vi "Gestione_Inverter.vi"(6 "Inverter":refnum<vi>, 7 "Stato rpm":refnum<vi>, 8 "Test settings":refnum<vi>, 9 "RS485":refnum<vi>, 10 "Cluster ALARMS":refnum<vi>, 11 "name":string) -> ()   [LabVIEW 2019]
uses:
  Letture inverter.ctl
  Parametri inverter.ctl
  Da TDE TestDrive/Tipi di parametro.ctl
  Set inverter.ctl
  <vilib>/Modbus/subvis/Modbus API/Modbus API.lvclass/Modbus API.ctl
  <vilib>/Modbus/subvis/Transmission Data Unit (ADU)/Transmission Data Unit/Transmission Data Unit.lvclass/Transmission Data Unit.ctl
  <vilib>/Modbus/master/Data Access/Unit ID/Set Unit ID Property.vi
  <vilib>/Modbus/subvis/Transmission Data Unit (ADU)/Transmission Data Unit/Data Access/Unit ID/Write Unit ID.vi
  <vilib>/Modbus/subvis/Modbus API/Read Transmission Data Unit.vi
  <vilib>/Modbus/subvis/Modbus API/Write Transmission Data Unit.vi
  <vilib>/Modbus/master/Modbus Master.lvclass
  C:/Program Files (x86)/National Instruments/LabVIEW 2019/vi.lib/Modbus/subvis/Modbus API/Modbus API.lvclass
  <vilib>/Utility/file.llb/Read From Spreadsheet File (string).vi
  <vilib>/Modbus/master/Create Master Instance (Serial).vi
  <vilib>/Modbus/subvis/Transmission Data Unit (ADU)/Transmission Data Unit/Transmission Data Unit.lvclass
panel:
  in  "SET INVERTER":bool
  in  "Test settings 2":T1 caption="PARAMETRI INVERTER"
  in  "Scelta inverter":T2(radio)=enum."INVERTER 1 \n[7,5kW]"
  out "id":u8
  in  "stop":bool
  out "DRIVE INOM":dbl
  out "Numeric":i32
  out "status":string
  out "output cluster":T3
  out "error out":errorcluster
  # "Caratteristiche motore"
  # "Limiti massimi"
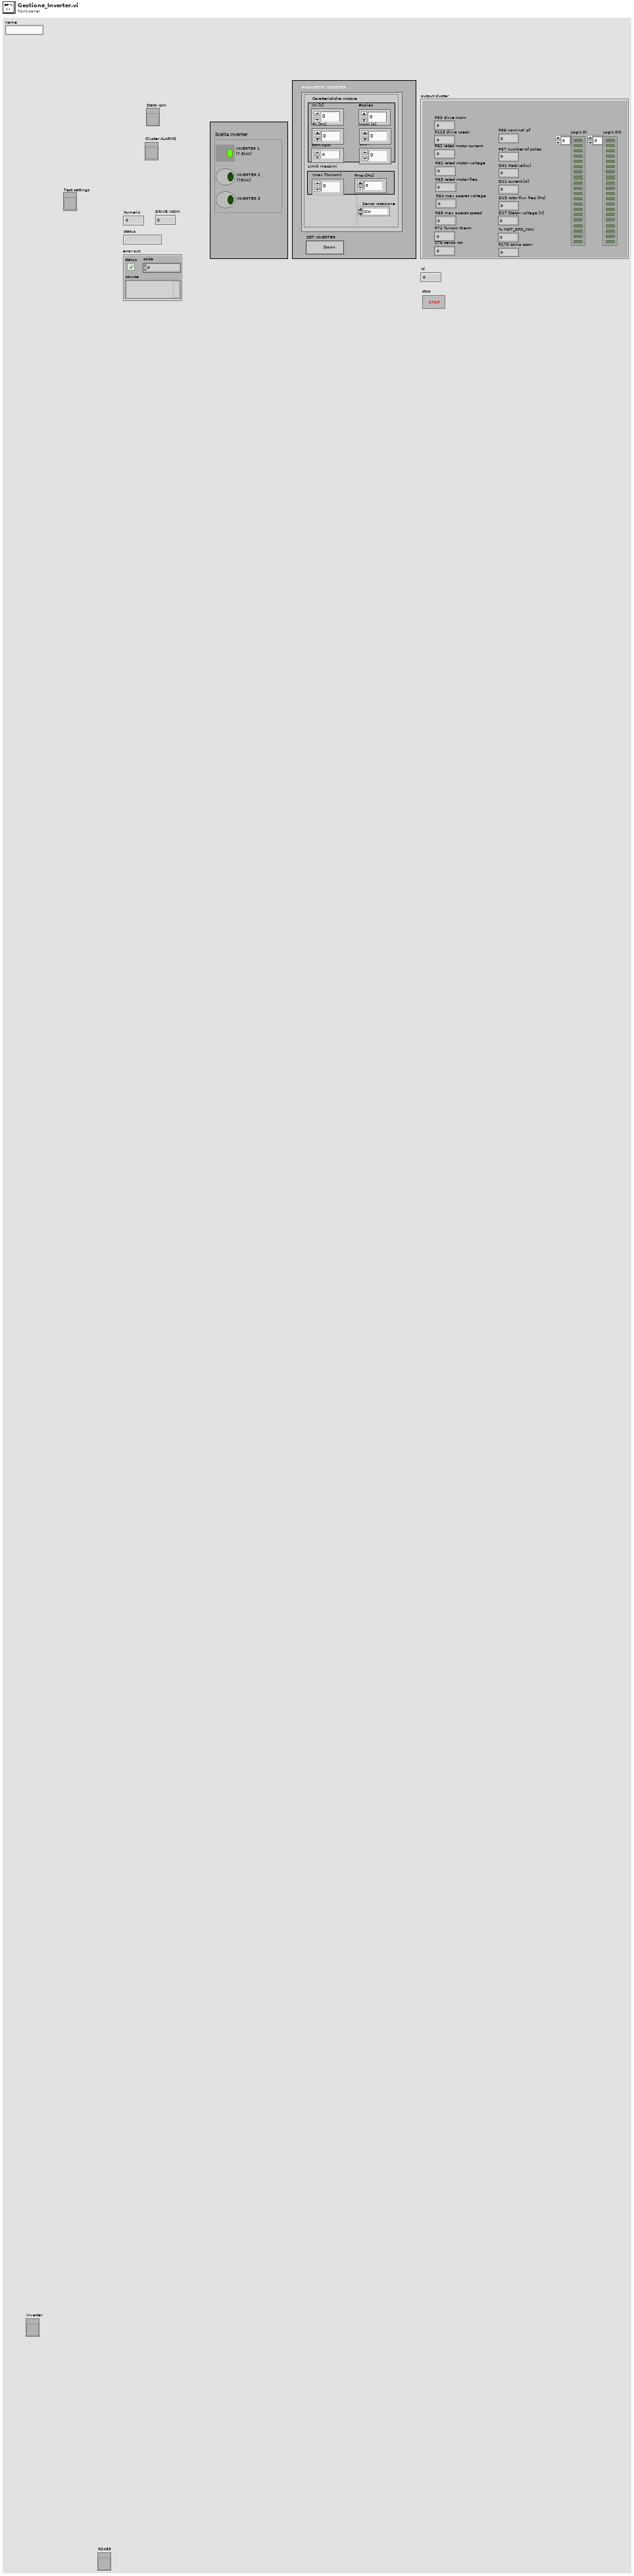
[diagram p1: front panel]
types:
  T1 = typedef "Parametri inverter.ctl" = cluster{"Vn [V]":dbl, "Fn [Hz]":dbl, "CosFi":dbl, "Imax [%Inom]":dbl, "#poles":dbl, "Inom [A]":dbl, "Senso rotazione":enum16{"CW", "CCW"}, "RPM nom":dbl, "Fmax[Hz]":dbl}
  T2 = enum32{"No Selection", "INVERTER 1 \n[7,5kW]", "INVERTER 2 \n[75kW]", "INVERTER 3"}
  T3 = typedef "Letture inverter.ctl" = cluster{"P61 rated motor current":dbl, "P62 rated motor voltage":dbl, "P63 rated motor freq":dbl, "P64 max operat voltage":dbl, "P65 max operat speed":dbl, "P66 nominal pf":dbl, "P67 number of poles":dbl, "D01 Pattiva[kw]":dbl, "D11 current [A]":dbl, "D13 rotor flux freq [Hz]":dbl, "D17 Stator voltage [V]":dbl, "% MOT_SPD_MAX":dbl, "Logic DI":bool[], "Logic DO":bool[], "P71 %inom therm":dbl, "P53 dirve Inom":dbl, "P113 dirve Ipeak":dbl, "C76 senso rot":dbl, "P170 comp scorr":dbl}
  T4 = typedef "Tipi di parametro.ctl" = u16
  T5 = typedef "Set inverter.ctl" = cluster{"F [Hz]":dbl}
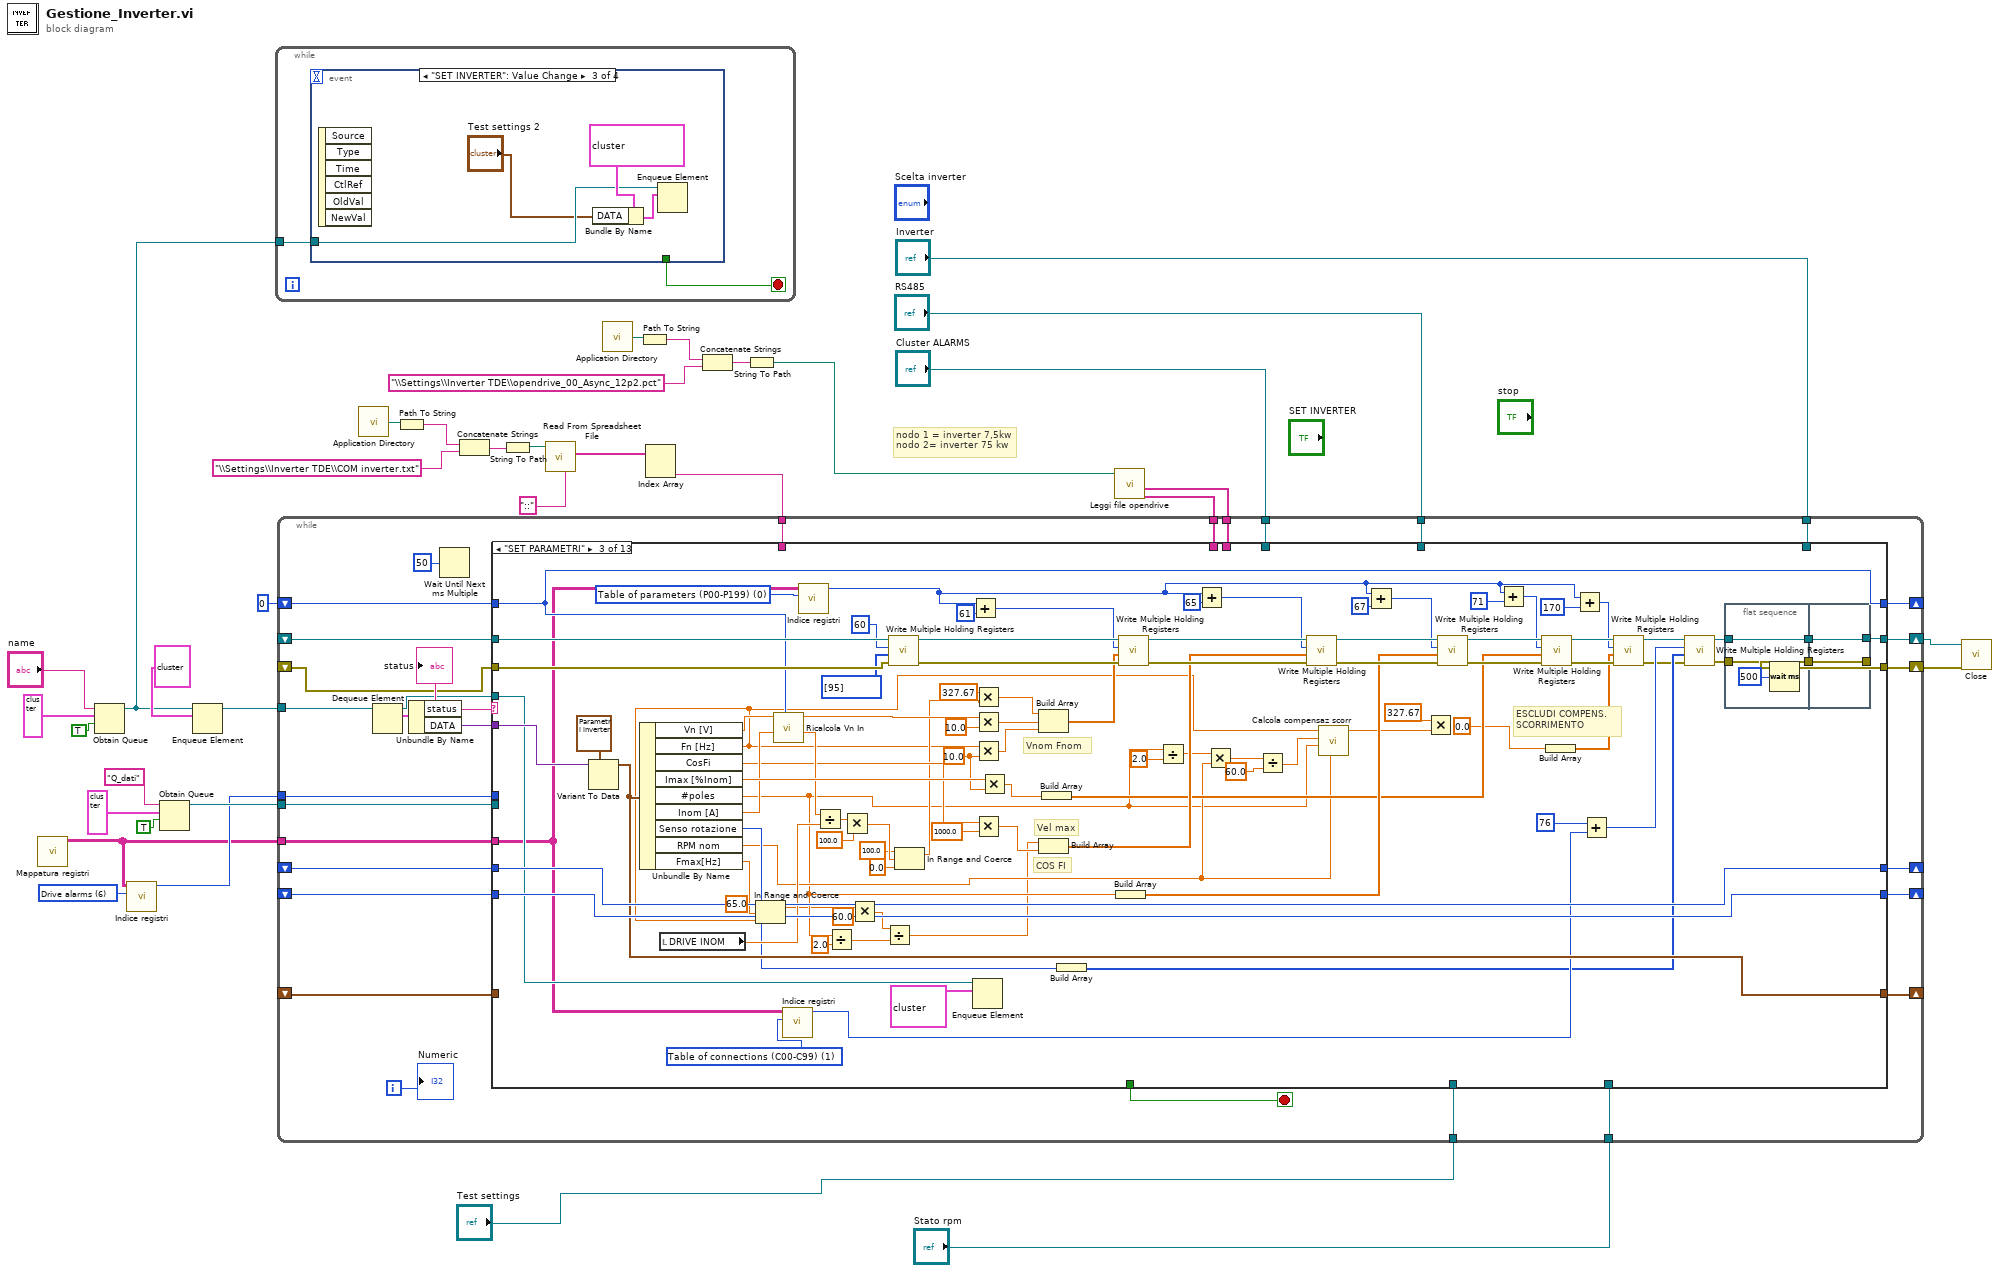
[diagram p0: block diagram]
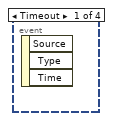
[diagram p2: hidden frame]
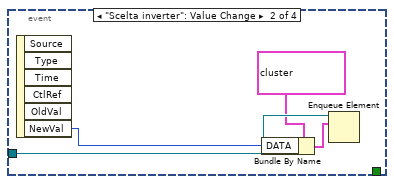
[diagram p3: hidden frame]
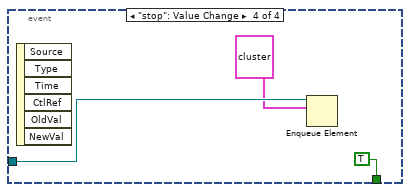
[diagram p4: hidden frame]
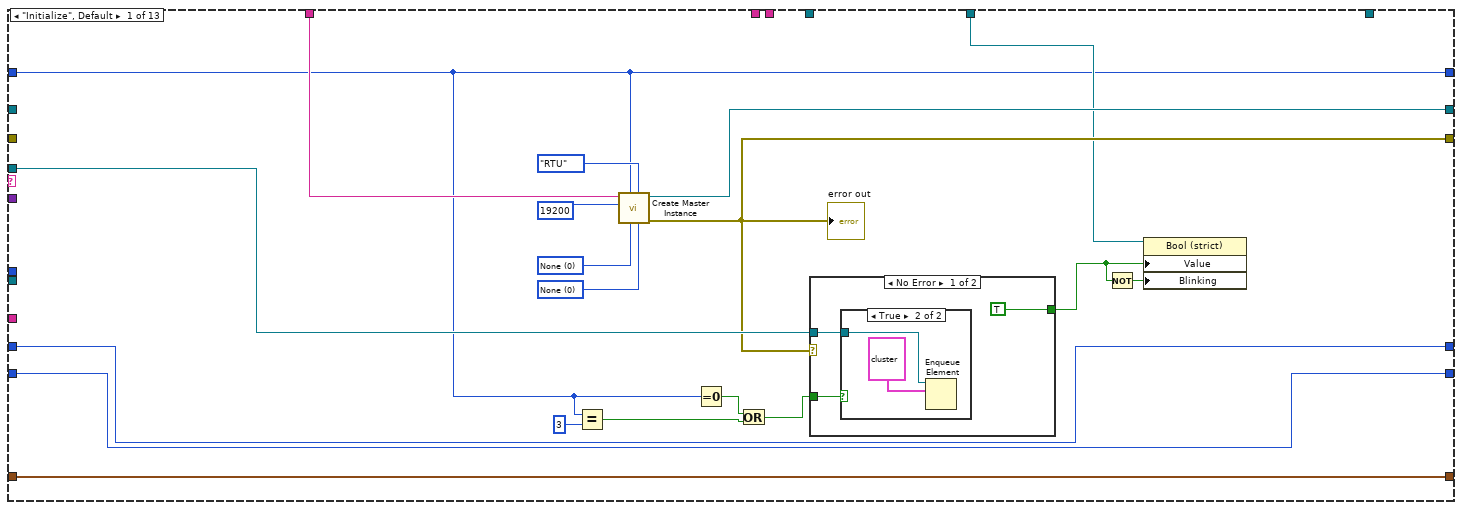
[diagram p5: hidden frame]
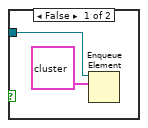
[diagram p6: hidden frame]
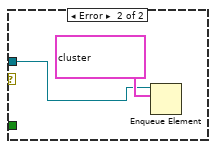
[diagram p7: hidden frame]
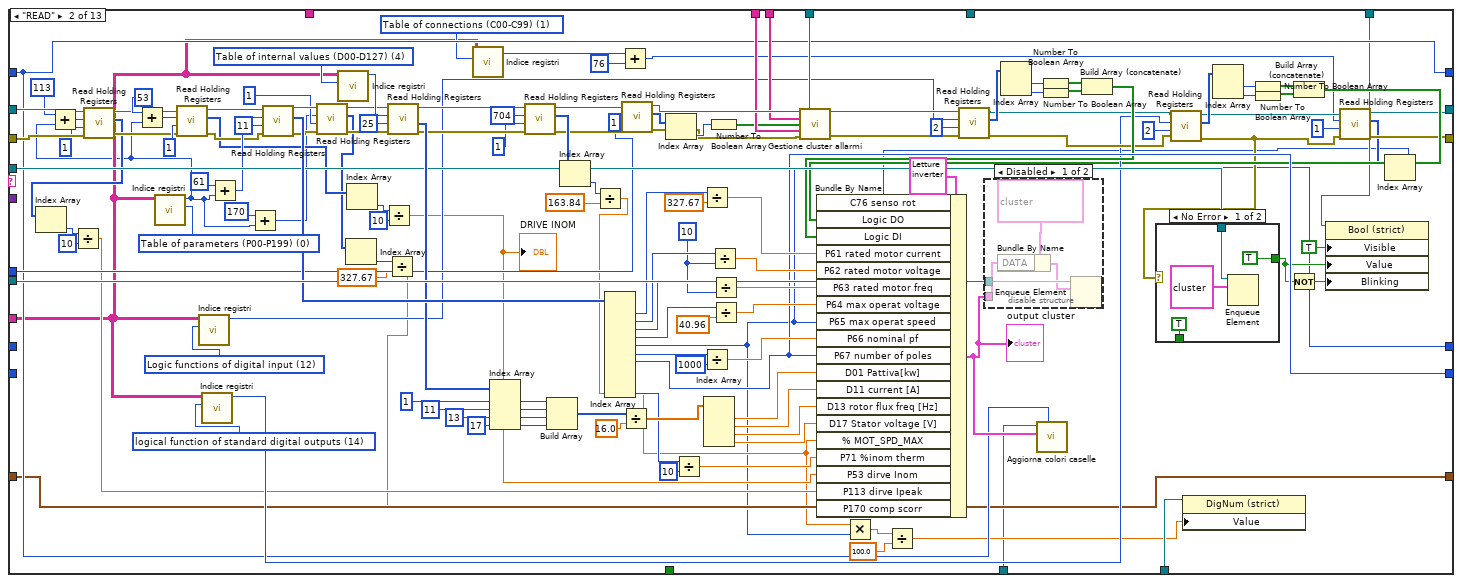
[diagram p8: hidden frame]
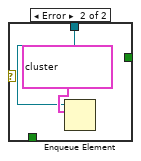
[diagram p10: hidden frame]
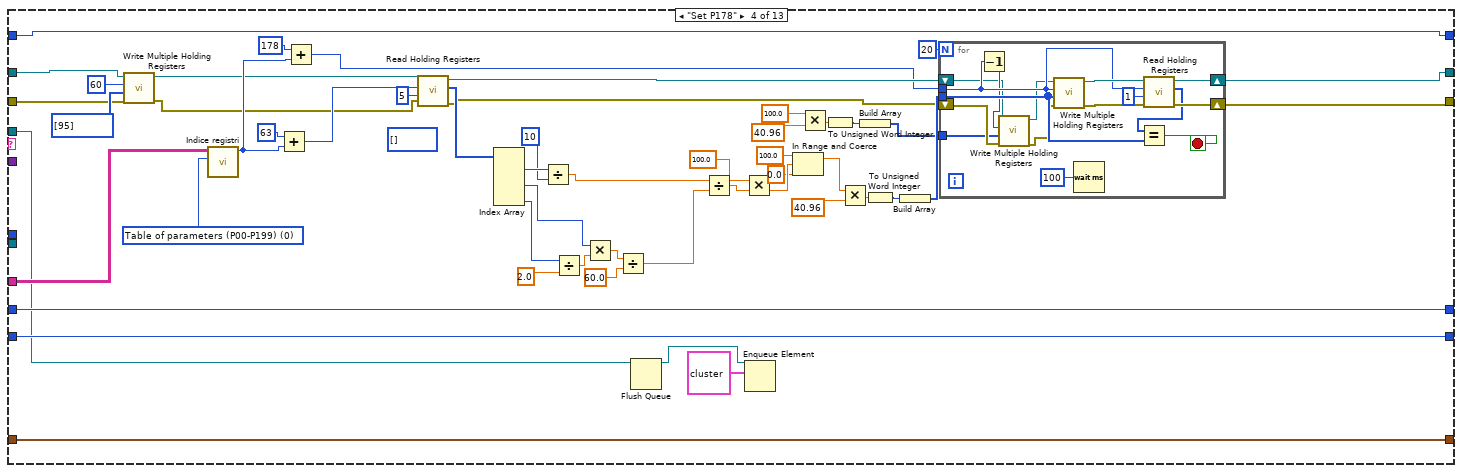
[diagram p11: hidden frame]
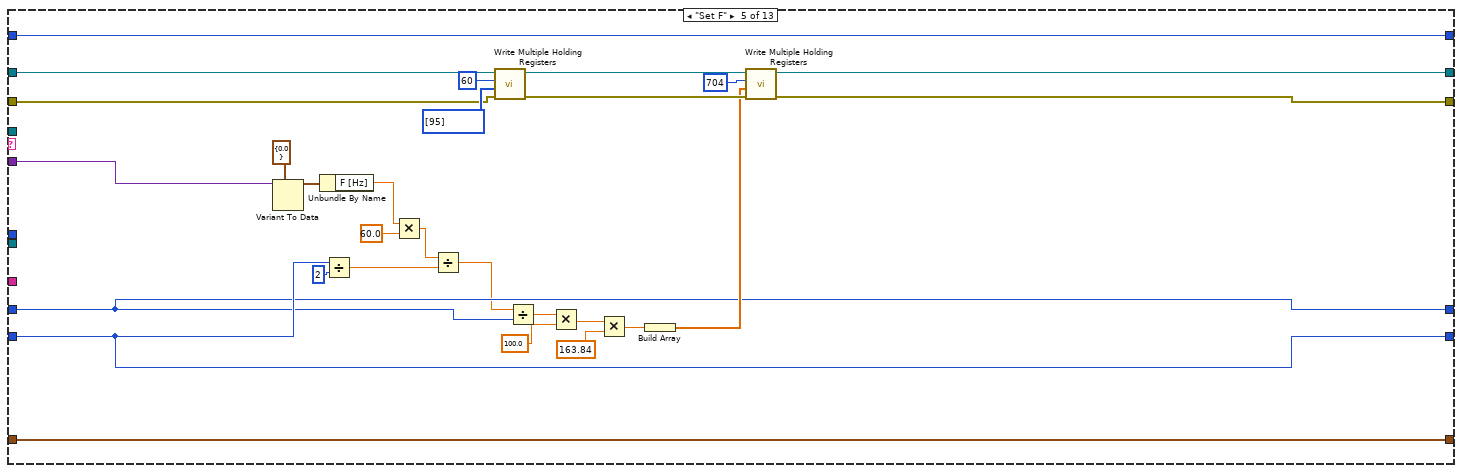
[diagram p12: hidden frame]
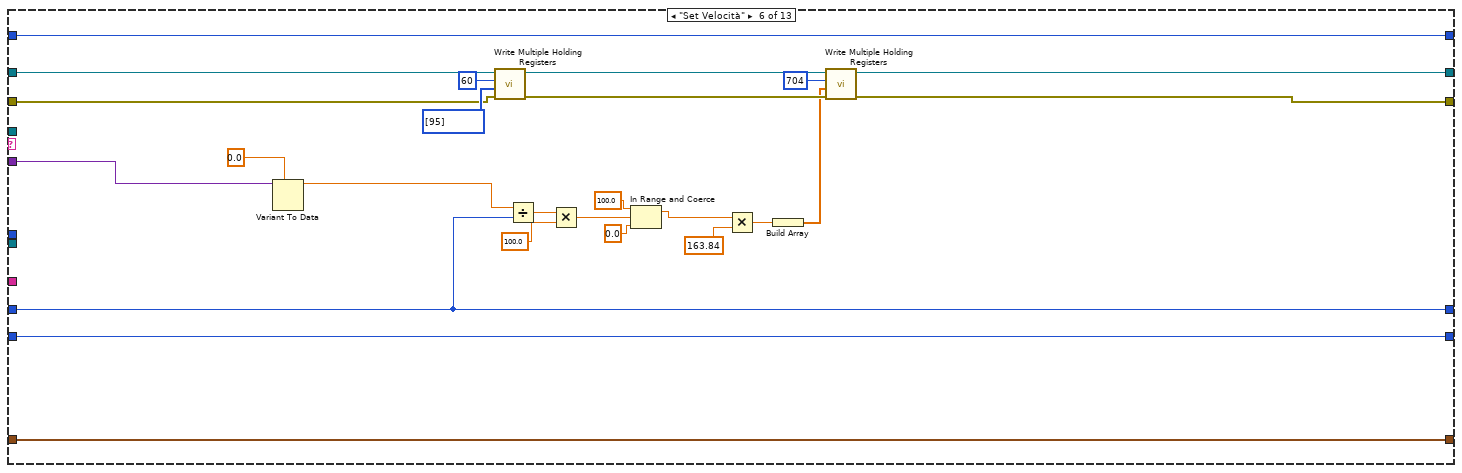
[diagram p13: hidden frame]
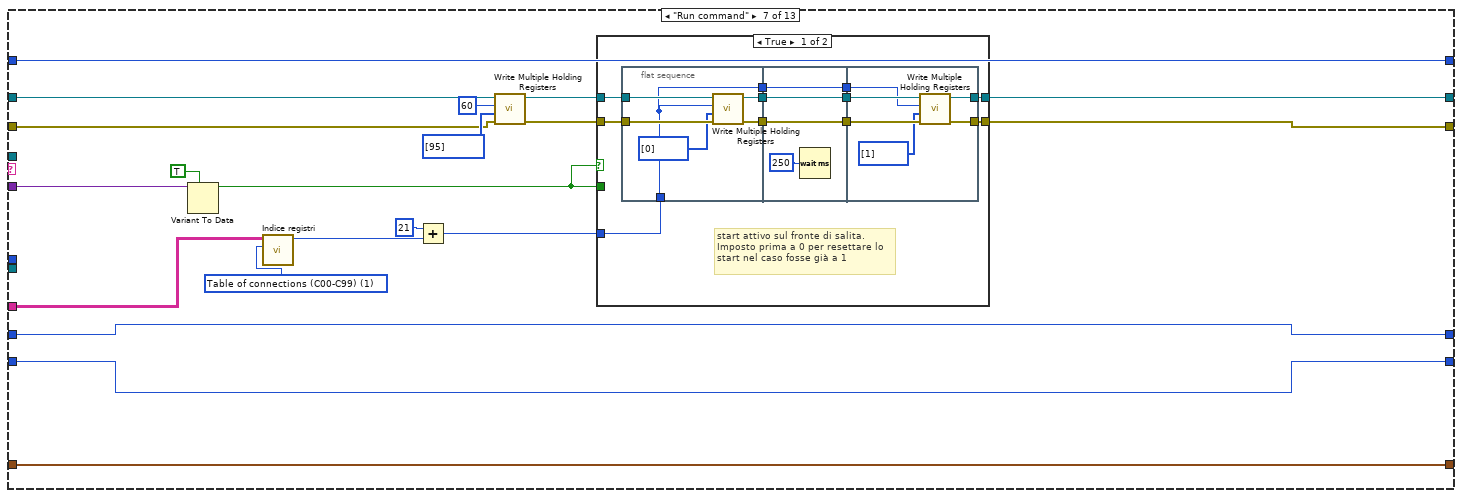
[diagram p14: hidden frame]
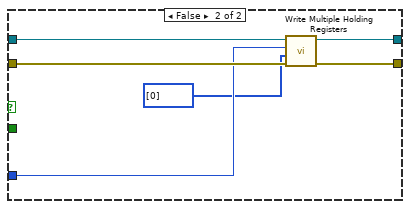
[diagram p15: hidden frame]
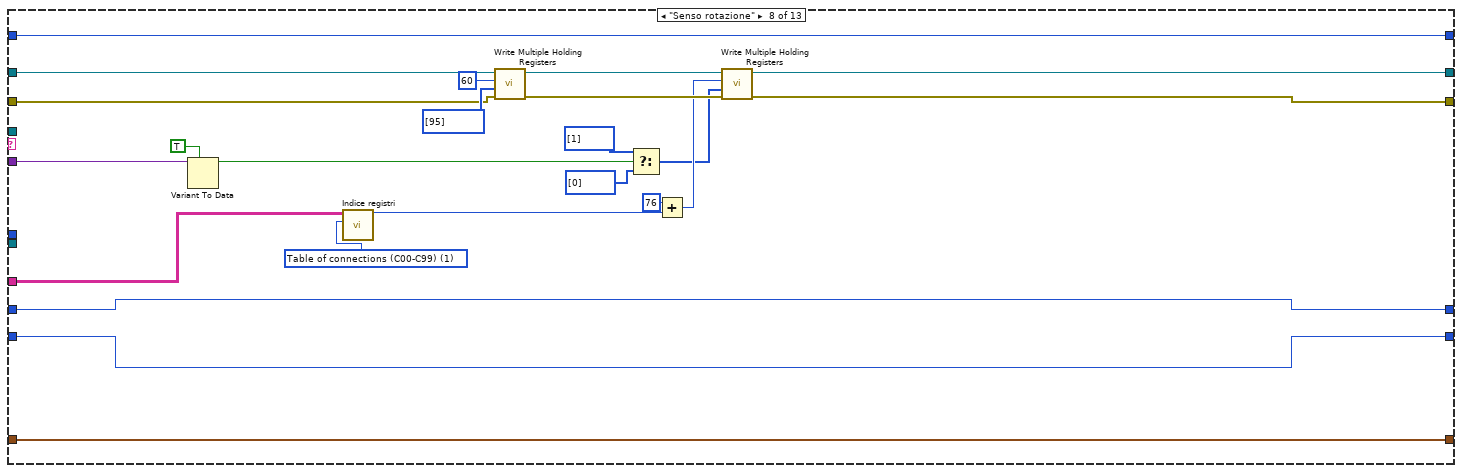
[diagram p16: hidden frame]
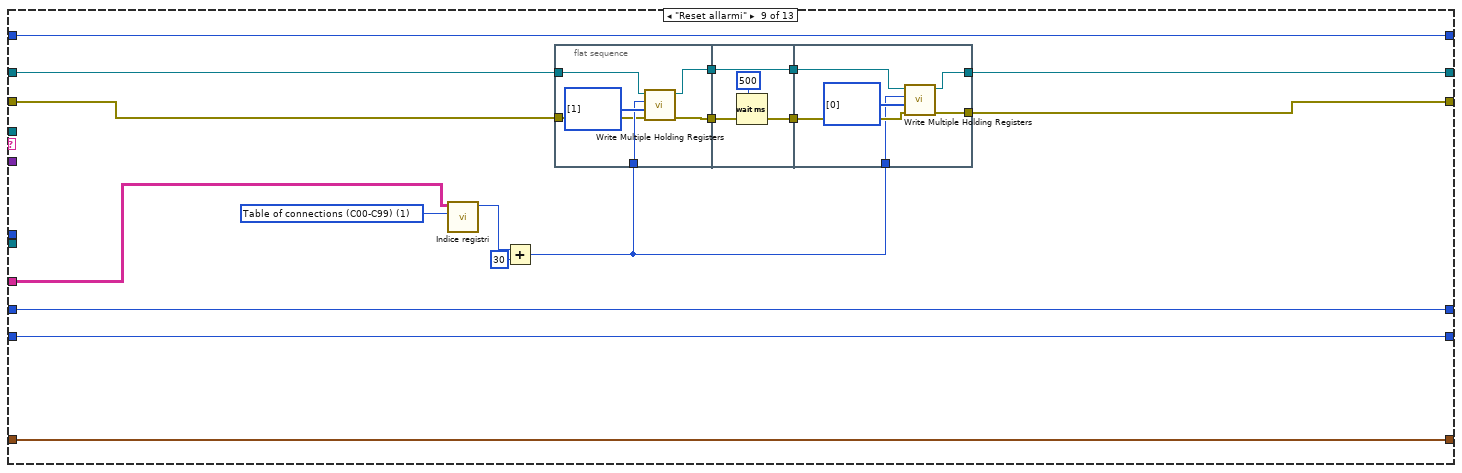
[diagram p17: hidden frame]
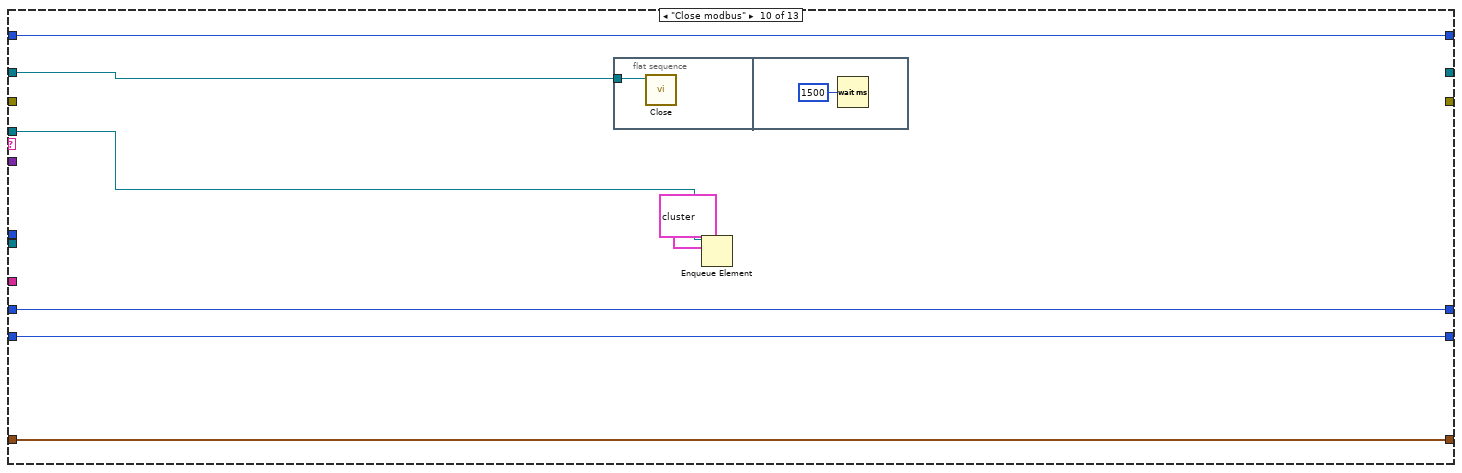
[diagram p18: hidden frame]
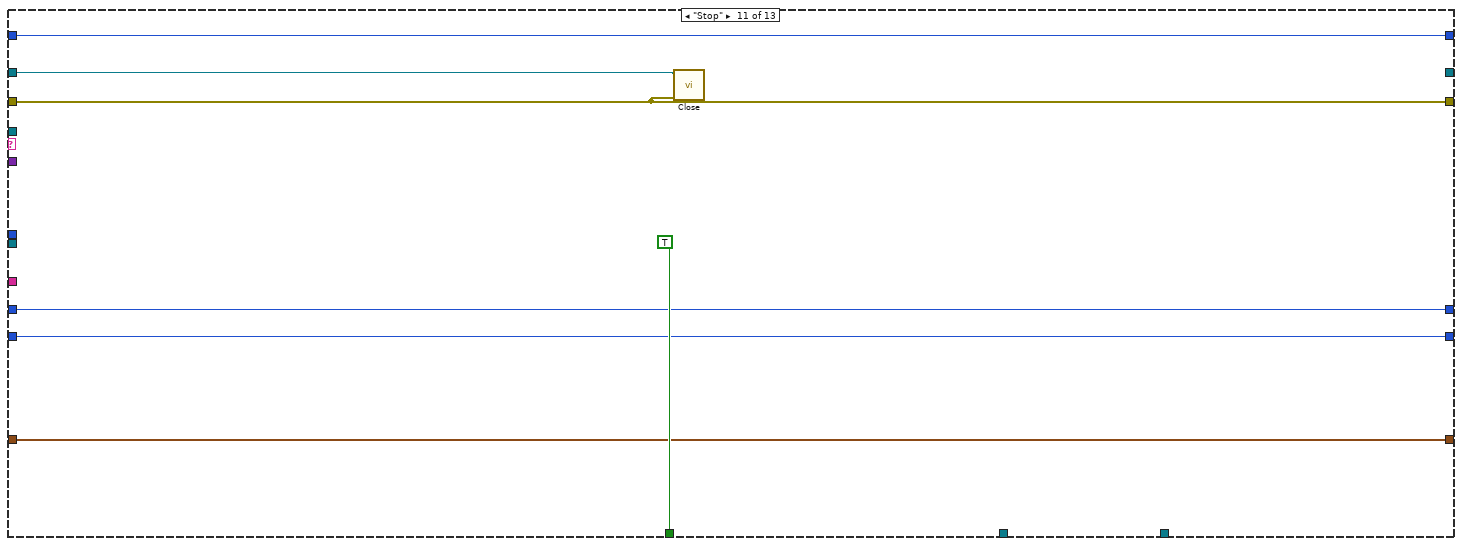
[diagram p19: hidden frame]
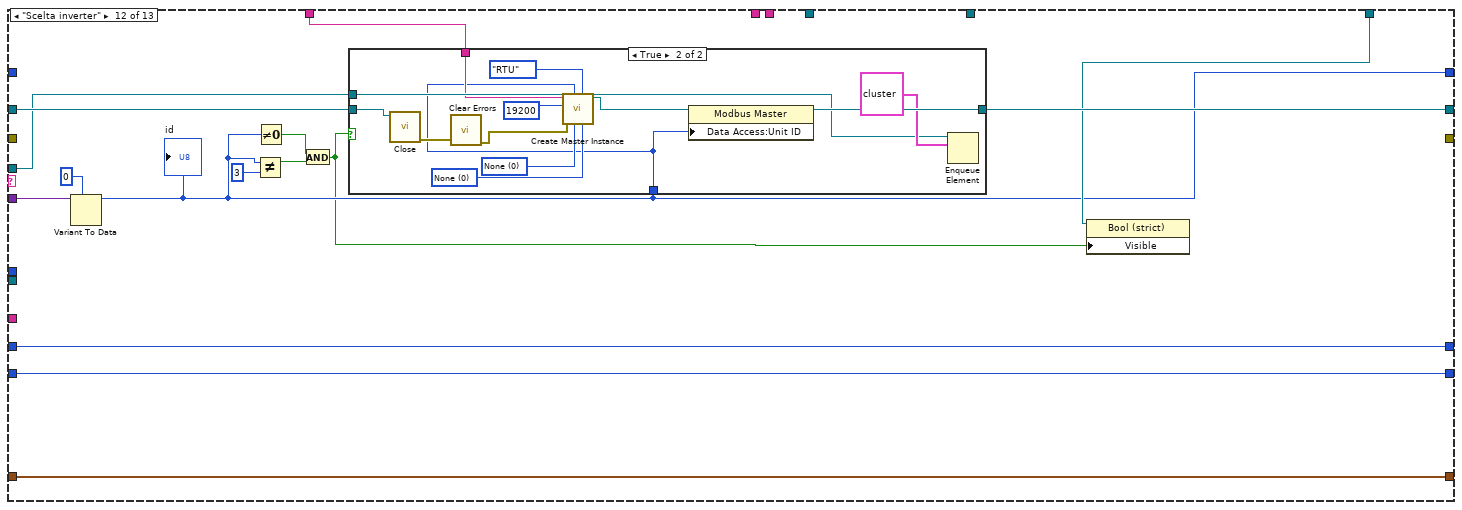
[diagram p20: hidden frame]
diagram:
  w25 = T4 6 items=["Table of parameters (P00-P199)", "Table of connections (C00-C99)", "Table of application parameters (E00-E99)", "Table of expanded application parameters (E100-E600)", "Table of internal values (D00-D127)", "Drive state", "Drive alarms", "Alarm enabling", "Speed reference from fieldbus", "Torque limit from fieldbus", "Torque reference from fieldbus", "Mechanical position read", "Logic functions of digital input", "Logic funtction of digital input from serial c.", "logical function of standard digital outputs", "logic function of application digital output", "Table of parameters formats", "Table of connections formats", "Table of monitor and analog outputs values", "Table of application parameters formats", "Table of internal values formats", "Scorta 1", "Scorta 2", "Scorta 3", "Scorta 4", "Scorta 5", "Scorta 6", "Scorta 7", "Scorta 8", "Scorta 9", "Scorta 10"] ("Lista tipi di parametro")
  # "nodo 1 = inverter 7,5kw\nnodo 2= inverter 75 kw"
  n1 = call "Mappatura registri.vi"() -> ("Mappa registri"=w20:string[][])  [unwired: 11 in]
  n2 = Obtain Queue(name (unnamed)="name", element data type=cluster{"DATA":variant, "status":string} {"DATA"=variant, "status"=""} ("output cluster"), create if not found? (T)=TRUE) -> (queue out=w5:refnum<queue>)  [unwired: 2 in, 2 out]
  n3 = call "Indice registri.vi"("Lista tipi di parametro"=w25, "Mappa registri"=w20) -> ("Registro iniziale"=w24:i32)  [unwired: 7 in, 2 out]
  n4 = Obtain Queue(name (unnamed)="Q_dati", element data type=cluster{"DATA":variant, "status":string} {"DATA"=variant, "status"=""} ("output cluster"), create if not found? (T)=TRUE) -> (queue out=w30:refnum<queue>)  [unwired: 2 in, 2 out]
  n5 = Enqueue Element(queue=w5, element=cluster{"DATA":variant, "status":string} {"DATA"=variant, "status"="IDLE"}) -> (queue out=w28:refnum<queue>)  [unwired: 2 in, 2 out]
  n6 = while {
    tunnel: w5 -> [w38]
    stop <- w37 stop-if-true
    n7 = event shown="[2] \"SET INVERTER\": Value Change" {
      selector: _ -> [_ _ _ _]
      dyn-events: _ -> [_ _ _ _]
      timeout: _ -> [_ _ _ _]
      tunnel: w38 -> [_ w42 w44 w49]
      tunnel: [_ _ _ TRUE] -> w37
      event Timeout {
        n8 = event-data() -> ()  [unwired: 1 in, 3 out]
      }
      event "Scelta inverter": Value Change {
        n9 = event-data() -> ("NewVal"=w39:T2)  [unwired: 1 in, 5 out]
        n10 = Bundle By Name(cluster=cluster{"DATA":variant, "status":string} {"DATA"=variant, "status"="Scelta inverter"} ("element"), "DATA"=w39) -> (w40:cluster{"DATA":variant, "status":string})
        n11 = Enqueue Element(queue=w42, element=w40) -> ()  [unwired: 2 in, 3 out]
      }
      event "SET INVERTER": Value Change {
        n12 = event-data() -> ()  [unwired: 1 in, 6 out]
        n13 = Bundle By Name(cluster=cluster{"DATA":variant, "status":string} {"DATA"=variant, "status"="SET PARAMETRI"} ("element"), "DATA"="Test settings 2") -> (w45:cluster{"DATA":variant, "status":string})
        n14 = Enqueue Element(queue=w44, element=w45) -> ()  [unwired: 2 in, 3 out]
      }
      event "stop": Value Change {
        n15 = event-data() -> ()  [unwired: 1 in, 6 out]
        n16 = Enqueue Element(queue=w49, element=cluster{"DATA":variant, "status":string} {"DATA"=variant, "status"="Stop"}) -> ()  [unwired: 2 in, 3 out]
      }
    }
  }
  n17 = call <vilib>:"Application Directory.vi"() -> ("Application Directory"=w14:path)
  n18 = Path To String(path=w14) -> (string=w15:string)
  n19 = Concatenate Strings(w15, "\\Settings\\Inverter TDE\\COM inverter.txt" ("name or relative path")) -> (w17:string)
  n20 = String To Path(string=w17) -> (path=w18:path)
  n21 = call-poly <vilib>:"Read From Spreadsheet File.vi"("delimiter (\\t)"="::" ("delimiter (\\t)"), "file path (dialog if empty)"=w18) -> ("first row"=w12:string[])  [unwired: 5 in, 4 out]
  n22 = call <vilib>:"Application Directory.vi"() -> ("Application Directory"=w10:path)
  n23 = Path To String(path=w10) -> (string=w9:string)
  n24 = Index Array(array=w12) -> (element #2=w11:string)  [unwired: 2 in, 1 out]
  n25 = Concatenate Strings(w9, "\\Settings\\Inverter TDE\\opendrive_00_Async_12p2.pct" ("name or relative path")) -> (w7:string)
  n26 = String To Path(string=w7) -> (path=w6:path)
  n27 = call "Leggi file opendrive.vi"("file path (dialog if empty)"=w6) -> ("Array descriz alarms"=w22:string[], "Array Name alarms"=w23:string[])  [unwired: 8 in, 1 out]
  n28 = while {
    tunnel: w28 -> [w80]
    shift-right: [w75] -> w26
    shift-left: _ -> [w52]
    shift-right: [w74] -> w27
    shift-left: _ -> [w56]
    tunnel: w30 -> [w73]
    shift-right: [w69] -> _
    shift-left: _ -> [w68]
    shift-right: [w67] -> _
    shift-left: _ -> [w66]
    tunnel: w24 -> [w65]
    tunnel: w23 -> [w64]
    tunnel: w22 -> [w63]
    tunnel: "Cluster ALARMS" -> [w62]
    tunnel: w20 -> [w61]
    tunnel: "RS485" -> [w60]
    tunnel: w11 -> [w59]
    shift-right: [w58] -> _
    shift-left: _ -> [w57]
    tunnel: "Test settings" -> [w55]
    shift-right: [w54] -> _
    shift-left: u8 0 ("unit ID") -> [w53]
    tunnel: "Inverter" -> [w51]
    tunnel: "Stato rpm" -> [w50]
    i -> [w70]
    stop <- w76 stop-if-true
    n29 = Dequeue Element(queue=w80) -> (queue out=w71:refnum<queue>, element=w79:cluster{"DATA":variant, "status":string})  [unwired: 2 in, 2 out]
    n30 = Unbundle By Name(w79) -> ("status"=w78:string, "DATA"=w77:variant)
    "status" <- w78
    n31 = Wait Until Next ms Multiple(millisecond multiple=u32 50) -> ()  [unwired: 1 out]
    n32 = case shown="\"SET PARAMETRI\"" w78 {
      tunnel: w77 -> [_ _ w357 _ w449 w474 w493 w549 _ _ _ w617 _]
      tunnel: [_ _ _ _ _ _ _ _ _ _ TRUE _ _] -> w76
      tunnel: [w99 w128 w317 w394 w451 w476 w497 w553 w567 _ _ w618 w641] -> w75
      tunnel: [w93 w126 w316 w395 w450 w475 w496 w552 w563 _ w605 _ w640] -> w74
      tunnel: w52 -> [_ w155 w356 w371 w453 w478 w499 w555 w570 w598 w606 w619 w641]
      tunnel: w56 -> [_ w157 w355 w369 w452 w477 w498 w554 w566 _ w605 _ w640]
      tunnel: w73 -> [_ w252 _ _ _ _ _ _ _ _ _ _ _]
      tunnel: w71 -> [w94 w217 w313 w363 _ _ _ _ _ w596 _ w615 _]
      tunnel: [w92 w110 w338 w414 w434 w466 w494 w550 w576 w595 w604 w622 w645] -> w69
      tunnel: w68 -> [w92 _ w338 w414 w434 w466 w494 w550 w576 w595 w604 w622 w645]
      tunnel: [w91 w216 w337 w413 w443 w473 w495 w551 w575 w594 w603 w621 w644] -> w67
      tunnel: w66 -> [w91 _ w337 w413 w443 w473 w495 w551 w575 w594 w603 w621 w644]
      tunnel: w65 -> [_ w198 _ _ _ _ _ _ _ _ _ _ _]
      tunnel: w64 -> [_ w205 _ _ _ _ _ _ _ _ _ _ _]
      tunnel: w63 -> [_ w204 _ _ _ _ _ _ _ _ _ _ _]
      tunnel: w62 -> [_ w200 _ _ _ _ _ _ _ _ _ _ _]
      tunnel: w61 -> [_ w133 w300 w411 _ _ w490 w546 w573 _ _ _ _]
      tunnel: w60 -> [w89 _ _ _ _ _ _ _ _ _ _ _ _]
      tunnel: w59 -> [w86 _ _ _ _ _ _ _ _ _ _ w608 _]
      tunnel: [w87 w144 w311 w367 w432 w465 w486 w538 w561 w593 w602 w620 w643] -> w58
      tunnel: w57 -> [w87 w144 _ w367 w432 w465 w486 w538 w561 w593 w602 w620 w643]
      tunnel: w53 -> [w84 w145 w306 w366 w431 w464 w485 w537 w560 w592 w601 _ w642]
      tunnel: w55 -> [_ w109 _ _ _ _ _ _ _ _ _ _ _]
      tunnel: [w84 w145 w306 w366 w431 w464 w485 w537 w560 w592 w601 w613 w642] -> w54
      tunnel: w51 -> [_ w141 _ _ _ _ _ _ _ _ _ w614 _]
      tunnel: w50 -> [_ w136 _ _ _ _ _ _ _ _ _ _ _]
      frame "Initialize", Default {
        w96 = u16 0 items=["None", "XON/XOFF", "RTS/CTS", "XON/XOFF & RTS/CTS", "DTR/DSR", "XON/XOFF & DTR/DSR"] ("flow control (None)")
        w97 = u16 0 items=["None", "Odd", "Even"] ("parity (Even)")
        n33 = Equal?(x=w84, y=u8 3) -> (x = y?=w82:bool)
        n34 = call-poly <vilib>:"Create Master Instance.vi"("flow control (None)"=w96, "serial type"=enum16{"RTU", "ASCII"}."RTU", "parity (Even)"=w97, "unit ID"=w84, "baud rate (9600)"=u32 19200, "VISA resource name"=w86) -> ("error out"=w93:errorcluster, "serial master instance"=w99:refnum<class "Modbus Master.lvclass">)  [unwired: 4 in]
        "error out" <- w93
        n35 = Equal To 0?(x=w84) -> (x = 0?=w85:bool)
        n36 = Or(x=w85, y=w82) -> (x .or. y?=w81:bool)
        n37 = case shown="No Error" w93 {
          tunnel: w94 -> [w102 w107]
          tunnel: [TRUE _] -> w88
          tunnel: w81 -> [w100 _]
          frame No Error {
            n38 = case shown="True" w100 {
              tunnel: w102 -> [w103 w106]
              frame False {
                n39 = Enqueue Element(queue=w103, element=cluster{"DATA":variant, "status":string} {"DATA"=variant, "status"="READ"}) -> ()  [unwired: 2 in, 3 out]
              }
              frame True {
                n40 = Enqueue Element(queue=w106, element=cluster{"DATA":variant, "status":string} {"DATA"=variant, "status"="IDLE"}) -> ()  [unwired: 2 in, 3 out]
              }
            }
          }
          frame Error {
            n41 = Enqueue Element(queue=w107, element=cluster{"DATA":variant, "status":string} {"DATA"=variant, "status"="Close modbus"}) -> ()  [unwired: 2 in, 3 out]
          }
        }
        n42 = Not(x=w88) -> (.not. x?=w90:bool)
        n43 = property class="Bool (strict)"(reference=w89, "Value"=w88, "Blinking"=w90) -> ()  [unwired: 1 in, 2 out]
      }
      frame "READ" {
        w134 = T4 1 items=["Table of parameters (P00-P199)", "Table of connections (C00-C99)", "Table of application parameters (E00-E99)", "Table of expanded application parameters (E100-E600)", "Table of internal values (D00-D127)", "Drive state", "Drive alarms", "Alarm enabling", "Speed reference from fieldbus", "Torque limit from fieldbus", "Torque reference from fieldbus", "Mechanical position read", "Logic functions of digital input", "Logic funtction of digital input from serial c.", "logical function of standard digital outputs", "logic function of application digital output", "Table of parameters formats", "Table of connections formats", "Table of monitor and analog outputs values", "Table of application parameters formats", "Table of internal values formats", "Scorta 1", "Scorta 2", "Scorta 3", "Scorta 4", "Scorta 5", "Scorta 6", "Scorta 7", "Scorta 8", "Scorta 9", "Scorta 10"] ("Lista tipi di parametro")
        w180 = T4 14 items=["Table of parameters (P00-P199)", "Table of connections (C00-C99)", "Table of application parameters (E00-E99)", "Table of expanded application parameters (E100-E600)", "Table of internal values (D00-D127)", "Drive state", "Drive alarms", "Alarm enabling", "Speed reference from fieldbus", "Torque limit from fieldbus", "Torque reference from fieldbus", "Mechanical position read", "Logic functions of digital input", "Logic funtction of digital input from serial c.", "logical function of standard digital outputs", "logic function of application digital output", "Table of parameters formats", "Table of connections formats", "Table of monitor and analog outputs values", "Table of application parameters formats", "Table of internal values formats", "Scorta 1", "Scorta 2", "Scorta 3", "Scorta 4", "Scorta 5", "Scorta 6", "Scorta 7", "Scorta 8", "Scorta 9", "Scorta 10"] ("Lista tipi di parametro")
        w191 = T4 12 items=["Table of parameters (P00-P199)", "Table of connections (C00-C99)", "Table of application parameters (E00-E99)", "Table of expanded application parameters (E100-E600)", "Table of internal values (D00-D127)", "Drive state", "Drive alarms", "Alarm enabling", "Speed reference from fieldbus", "Torque limit from fieldbus", "Torque reference from fieldbus", "Mechanical position read", "Logic functions of digital input", "Logic funtction of digital input from serial c.", "logical function of standard digital outputs", "logic function of application digital output", "Table of parameters formats", "Table of connections formats", "Table of monitor and analog outputs values", "Table of application parameters formats", "Table of internal values formats", "Scorta 1", "Scorta 2", "Scorta 3", "Scorta 4", "Scorta 5", "Scorta 6", "Scorta 7", "Scorta 8", "Scorta 9", "Scorta 10"] ("Lista tipi di parametro")
        w193 = T4 4 items=["Table of parameters (P00-P199)", "Table of connections (C00-C99)", "Table of application parameters (E00-E99)", "Table of expanded application parameters (E100-E600)", "Table of internal values (D00-D127)", "Drive state", "Drive alarms", "Alarm enabling", "Speed reference from fieldbus", "Torque limit from fieldbus", "Torque reference from fieldbus", "Mechanical position read", "Logic functions of digital input", "Logic funtction of digital input from serial c.", "logical function of standard digital outputs", "logic function of application digital output", "Table of parameters formats", "Table of connections formats", "Table of monitor and analog outputs values", "Table of application parameters formats", "Table of internal values formats", "Scorta 1", "Scorta 2", "Scorta 3", "Scorta 4", "Scorta 5", "Scorta 6", "Scorta 7", "Scorta 8", "Scorta 9", "Scorta 10"] ("Lista tipi di parametro")
        w196 = T4 0 items=["Table of parameters (P00-P199)", "Table of connections (C00-C99)", "Table of application parameters (E00-E99)", "Table of expanded application parameters (E100-E600)", "Table of internal values (D00-D127)", "Drive state", "Drive alarms", "Alarm enabling", "Speed reference from fieldbus", "Torque limit from fieldbus", "Torque reference from fieldbus", "Mechanical position read", "Logic functions of digital input", "Logic funtction of digital input from serial c.", "logical function of standard digital outputs", "logic function of application digital output", "Table of parameters formats", "Table of connections formats", "Table of monitor and analog outputs values", "Table of application parameters formats", "Table of internal values formats", "Scorta 1", "Scorta 2", "Scorta 3", "Scorta 4", "Scorta 5", "Scorta 6", "Scorta 7", "Scorta 8", "Scorta 9", "Scorta 10"] ("Lista tipi di parametro")
        w238 = u16 10 ("x")
        n44 = call "Indice registri.vi"("Lista tipi di parametro"=w196, "Mappa registri"=w133) -> ("Registro iniziale"=w116:i32)  [unwired: 7 in, 2 out]
        n45 = Add(x=113, y=w116) -> (x+y=w153:i32)
        n46 = call-dynamic "Read Holding Registers.vi"("error in (no error)"=w157, "number of holding registers"=u16 1, "starting address"=w153, "Modbus master in"=w155) -> ("error out"=w156:errorcluster, "register values"=w148:u16[], "Modbus master out"=w154:refnum<class "Modbus Master.lvclass">)  [unwired: 5 in]
        n47 = Index Array(array=w148) -> (element=w149:u16)  [unwired: 1 in]
        n48 = Divide(x=w149, y=u16 10) -> (x/y=w147:dbl)
        n49 = Add(x=53, y=w116) -> (x+y=w163:i32)
        n50 = call-dynamic "Read Holding Registers.vi"("error in (no error)"=w156, "number of holding registers"=u16 1, "starting address"=w163, "Modbus master in"=w154) -> ("error out"=w165:errorcluster, "register values"=w161:u16[], "Modbus master out"=w166:refnum<class "Modbus Master.lvclass">)  [unwired: 5 in]
        n51 = call "Indice registri.vi"("Lista tipi di parametro"=w191, "Mappa registri"=w133) -> ("Registro iniziale"=w187:i32)  [unwired: 7 in, 2 out]
        n52 = call "Indice registri.vi"("Lista tipi di parametro"=w180, "Mappa registri"=w133) -> ("Registro iniziale"=w171:i32)  [unwired: 7 in, 2 out]
        n53 = Add(x=61, y=w116) -> (x+y=w194:i32)
        n54 = Add(x=170, y=w116) -> (x+y=w115:i32)
        n55 = call-dynamic "Read Holding Registers.vi"("error in (no error)"=w165, "number of holding registers"=u16 11, "starting address"=w194, "Modbus master in"=w166) -> ("error out"=w120:errorcluster, "register values"=w249:u16[], "Modbus master out"=w122:refnum<class "Modbus Master.lvclass">)  [unwired: 5 in]
        n56 = call-dynamic "Read Holding Registers.vi"("error in (no error)"=w120, "number of holding registers"=u16 1, "starting address"=w115, "Modbus master in"=w122) -> ("error out"=w119:errorcluster, "register values"=w114:u16[], "Modbus master out"=w121:refnum<class "Modbus Master.lvclass">)  [unwired: 5 in]
        n57 = call "Indice registri.vi"("Lista tipi di parametro"=w193, "Mappa registri"=w133) -> ("Registro iniziale"=w192:i32)  [unwired: 7 in, 2 out]
        n58 = Index Array(array=w114) -> (element=w113:u16)  [unwired: 1 in]
        n59 = Index Array(array=w161) -> (element=w160:u16)  [unwired: 1 in]
        n60 = Divide(x=w160, y=u16 10) -> (x/y=w158:dbl)
        "DRIVE INOM" <- w158
        n61 = Divide(x=w113, y=327.67) -> (x/y=w111:dbl)
        n62 = call-dynamic "Read Holding Registers.vi"("error in (no error)"=w119, "number of holding registers"=u16 25, "starting address"=w192, "Modbus master in"=w121) -> ("error out"=w215:errorcluster, "register values"=w233:u16[], "Modbus master out"=w214:refnum<class "Modbus Master.lvclass">)  [unwired: 5 in]
        n63 = call "Indice registri.vi"("Lista tipi di parametro"=w134, "Mappa registri"=w133) -> ("Registro iniziale"=w132:i32)  [unwired: 7 in, 2 out]
        n64 = Index Array(array=w233, index #1=1 ("index"), index #2=11 ("index"), index #3=13 ("index"), index #4=17 ("index")) -> (element #1=w228:u16, element #2=w227:u16, element #3=w226:u16, element #4=w225:u16)
        n65 = call-dynamic "Read Holding Registers.vi"("error in (no error)"=w215, "number of holding registers"=u16 1, "starting address"=u16 704, "Modbus master in"=w214) -> ("error out"=w208:errorcluster, "register values"=w211:u16[], "Modbus master out"=w207:refnum<class "Modbus Master.lvclass">)  [unwired: 5 in]
        n66 = Build Array(w228, w227, w226, w225) -> (w224:u16[])
        n67 = Index Array(array=w211) -> (element=w210:u16)  [unwired: 1 in]
        n68 = Divide(x=w210, y=163.84) -> (x/y=w139:dbl)
        n69 = Index Array(array=w249) -> (element #1=w243:u16, element #2=w241:u16, element #3=w239:u16, element #4=w236:u16, element #5=w110:u16, element #6=w235:u16, element #7=w216:u16, element #11=w169:u16)  [unwired: 11 in, 3 out]
        n70 = Add(x=w132, y=76) -> (x+y=w125:i32)
        n71 = Divide(x=w224, y=16.0) -> (x/y=w222:dbl[])
        n72 = call-dynamic "Read Holding Registers.vi"("error in (no error)"=w208, "number of holding registers"=u16 1 ("starting address"), "starting address"=w198, "Modbus master in"=w207) -> ("error out"=w199:errorcluster, "register values"=w203:u16[], "Modbus master out"=w206:refnum<class "Modbus Master.lvclass">)  [unwired: 5 in]
        n73 = Index Array(array=w203) -> (element=w202:u16)  [unwired: 1 in]
        n74 = Divide(x=w169, y=u16 10) -> (x/y=w167:dbl)
        n75 = Divide(x=w243, y=327.67) -> (x/y=w248:dbl)
        n76 = Divide(x=w235, y=u16 1000) -> (x/y=w244:dbl)
        n77 = Index Array(array=w222) -> (element #1=w221:dbl, element #2=w220:dbl, element #3=w219:dbl, element #4=w218:dbl)  [unwired: 4 in]
        n78 = Number To Boolean Array(number=w202) -> (Boolean array=w201:bool[])
        n79 = Divide(x=w241, y=w238) -> (x/y=w240:dbl)
        n80 = Divide(x=w239, y=w238) -> (x/y=w247:dbl)
        n81 = Divide(x=w236, y=40.96) -> (x/y=w246:dbl)
        n82 = call "Gestione cluster allarmi.vi"("serial master instance"=w206, "Cluster ALARMS"=w200, "Array Name alarms"=w205, "Boolean array"=w201, "Array descriz alarms"=w204, "error in (no error)"=w199) -> ("Modbus master out"=w189:refnum<class "Modbus Master.lvclass">, "error out"=w188:errorcluster)  [unwired: 8 in]
        n83 = Multiply(x=w139, y=w110) -> (x*y=w138:dbl)
        n84 = Divide(x=w138, y=100.0) -> (x/y=w135:dbl)
        n85 = call-dynamic "Read Holding Registers.vi"("error in (no error)"=w188, "number of holding registers"=u16 2 ("starting address"), "starting address"=w187, "Modbus master in"=w189) -> ("error out"=w172:errorcluster, "register values"=w186:u16[], "Modbus master out"=w173:refnum<class "Modbus Master.lvclass">)  [unwired: 5 in]
        n86 = Index Array(array=w186) -> (element #1=w185:u16, element #2=w184:u16)  [unwired: 2 in]
        n87 = Number To Boolean Array(number=w185) -> (Boolean array=w183:bool[])
        n88 = Number To Boolean Array(number=w184) -> (Boolean array=w182:bool[])
        n89 = Build Array (concatenate)(w183, w182) -> (w181:bool[])
        n90 = call-dynamic "Read Holding Registers.vi"("error in (no error)"=w172, "number of holding registers"=u16 2 ("starting address"), "starting address"=w171, "Modbus master in"=w173) -> ("error out"=w127:errorcluster, "register values"=w175:u16[], "Modbus master out"=w129:refnum<class "Modbus Master.lvclass">)  [unwired: 5 in]
        n91 = case shown="No Error" w127 {
          tunnel: w217 -> [w259 w261]
          tunnel: [TRUE _] -> _
          tunnel: [TRUE _] -> w142
          frame No Error {
            n92 = Enqueue Element(queue=w259, element=cluster{"DATA":variant, "status":string} {"DATA"=variant, "status"="READ"}) -> ()  [unwired: 2 in, 3 out]
          }
          frame Error {
            n93 = Enqueue Element(queue=w261, element=cluster{"DATA":variant, "status":string} {"DATA"=variant, "status"="Close modbus"}) -> ()  [unwired: 2 in, 3 out]
          }
        }
        n94 = property class="DigNum (strict)"(reference=w136, "Value"=w135) -> ()  [unwired: 1 in, 2 out]
        n95 = Index Array(array=w175) -> (element #1=w176:u16, element #2=w177:u16)  [unwired: 2 in]
        n96 = Number To Boolean Array(number=w176) -> (Boolean array=w178:bool[])
        n97 = Number To Boolean Array(number=w177) -> (Boolean array=w179:bool[])
        n98 = Not(x=w142) -> (.not. x?=w143:bool)
        n99 = Build Array (concatenate)(w178, w179) -> (w170:bool[])
        n100 = property class="Bool (strict)"(reference=w141, "Visible"=TRUE, "Value"=w142, "Blinking"=w143) -> ()  [unwired: 1 in, 2 out]
        n101 = call-dynamic "Read Holding Registers.vi"("error in (no error)"=w127, "number of holding registers"=u16 1 ("starting address"), "starting address"=w125, "Modbus master in"=w129) -> ("error out"=w126:errorcluster, "register values"=w124:u16[], "Modbus master out"=w128:refnum<class "Modbus Master.lvclass">)  [unwired: 5 in]
        n102 = Index Array(array=w124) -> (element=w123:u16)  [unwired: 1 in]
        n103 = Bundle By Name(cluster=T3 {"P61 rated motor current"=0.0, "P62 rated motor voltage"=0.0, "P63 rated motor freq"=0.0, "P64 max operat voltage"=0.0, "P65 max operat speed"=0.0, "P66 nominal pf"=0.0, "P67 number of poles"=0.0, "D01 Pattiva[kw]"=0.0, "D11 current [A]"=0.0, "D13 rotor flux freq [Hz]"=0.0, "D17 Stator voltage [V]"=0.0, "% MOT_SPD_MAX"=0.0, "Logic DI"=[], "Logic DO"=[], "P71 %inom therm"=0.0, "P53 dirve Inom"=0.0, "P113 dirve Ipeak"=0.0, "C76 senso rot"=0.0, "P170 comp scorr"=0.0} ("Letture inverter"), "C76 senso rot"=w123, "Logic DO"=w170, "Logic DI"=w181, "P61 rated motor current"=w248, "P62 rated motor voltage"=w240, "P63 rated motor freq"=w247, "P64 max operat voltage"=w246, "P65 max operat speed"=w110, "P66 nominal pf"=w244, "P67 number of poles"=w216, "D01 Pattiva[kw]"=w221, "D11 current [A]"=w220, "D13 rotor flux freq [Hz]"=w219, "D17 Stator voltage [V]"=w218, "% MOT_SPD_MAX"=w139, "P71 %inom therm"=w167, "P53 dirve Inom"=w158, "P113 dirve Ipeak"=w147, "P170 comp scorr"=w111) -> (w146:T3)
        "output cluster" <- w146
        n104 = disable-structure shown="Disabled" {
          disable-tunnel: w252 -> [w256 _]
          disable-tunnel: w146 -> [w253 _]
          frame Disabled {
            n105 = Bundle By Name(cluster=cluster{"DATA":variant, "status":string} {"DATA"=variant, "status"="Leggi inverter"} ("element"), "DATA"=w253) -> (w255:cluster{"DATA":variant, "status":string})
            n106 = Enqueue Element(queue=w256, element=w255) -> ()  [unwired: 2 in, 3 out]
          }
          frame Enabled {
          }
        }
        n107 = call "Aggiorna colori caselle.vi"("id"=w145, "Letture inverter"=w146, "Test settings"=w109) -> ()  [unwired: 9 in]
      }
      frame "SET PARAMETRI" {
        w301 = T4 1 items=["Table of parameters (P00-P199)", "Table of connections (C00-C99)", "Table of application parameters (E00-E99)", "Table of expanded application parameters (E100-E600)", "Table of internal values (D00-D127)", "Drive state", "Drive alarms", "Alarm enabling", "Speed reference from fieldbus", "Torque limit from fieldbus", "Torque reference from fieldbus", "Mechanical position read", "Logic functions of digital input", "Logic funtction of digital input from serial c.", "logical function of standard digital outputs", "logic function of application digital output", "Table of parameters formats", "Table of connections formats", "Table of monitor and analog outputs values", "Table of application parameters formats", "Table of internal values formats", "Scorta 1", "Scorta 2", "Scorta 3", "Scorta 4", "Scorta 5", "Scorta 6", "Scorta 7", "Scorta 8", "Scorta 9", "Scorta 10"] ("Lista tipi di parametro")
        w334 = T4 0 items=["Table of parameters (P00-P199)", "Table of connections (C00-C99)", "Table of application parameters (E00-E99)", "Table of expanded application parameters (E100-E600)", "Table of internal values (D00-D127)", "Drive state", "Drive alarms", "Alarm enabling", "Speed reference from fieldbus", "Torque limit from fieldbus", "Torque reference from fieldbus", "Mechanical position read", "Logic functions of digital input", "Logic funtction of digital input from serial c.", "logical function of standard digital outputs", "logic function of application digital output", "Table of parameters formats", "Table of connections formats", "Table of monitor and analog outputs values", "Table of application parameters formats", "Table of internal values formats", "Scorta 1", "Scorta 2", "Scorta 3", "Scorta 4", "Scorta 5", "Scorta 6", "Scorta 7", "Scorta 8", "Scorta 9", "Scorta 10"] ("Lista tipi di parametro")
        w320 = 10.0 ("y")
        # "ESCLUDI COMPENS.\nSCORRIMENTO"
        # "COS FI"
        # "Vel max"
        # "Vnom Fnom"
        n108 = Variant To Data(type=T1 {"Vn [V]"=400.0, "Fn [Hz]"=50.0, "CosFi"=65.0, "Imax [%Inom]"=65.0, "#poles"=4.0, "Inom [A]"=0.0, "Senso rotazione"=enum."CW", "RPM nom"=0.0, "Fmax[Hz]"=0.0} ("Test settings"), Variant=w357) -> (data=w311:T1)  [unwired: 1 in, 1 out]
        n109 = Unbundle By Name(w311) -> ("Vn [V]"=w349:dbl, "Fn [Hz]"=w265:dbl, "CosFi"=w286:dbl, "Imax [%Inom]"=w323:dbl, "#poles"=w268:dbl, "Inom [A]"=w309:dbl, "Senso rotazione"=w298:enum16{"CW", "CCW"}, "RPM nom"=w274:dbl, "Fmax[Hz]"=w269:dbl)
        n110 = local read "DRIVE INOM"() -> (w319:dbl)
        n111 = In Range and Coerce(upper limit=65.0, x=w269, lower limit=w265) -> (coerced(x)=w266:dbl)  [unwired: 1 out]
        n112 = call "Ricalcola Vn In.vi"("id"=w306, "In [A]"=w309, "Vn [V]"=w349) -> ("In out"=w307:dbl, "Vn out"=w310:dbl)  [unwired: 7 in]
        n113 = call "Indice registri.vi"("Lista tipi di parametro"=w301, "Mappa registri"=w300) -> ("Registro iniziale"=w299:i32)  [unwired: 7 in, 2 out]
        n114 = call "Indice registri.vi"("Lista tipi di parametro"=w334, "Mappa registri"=w300) -> ("Registro iniziale"=w292:i32)  [unwired: 7 in, 2 out]
        n115 = Divide(x=w307, y=w319) -> (x/y=w308:dbl)
        n116 = Divide(x=w268, y=2.0) -> (x/y=w273:dbl)
        n117 = Multiply(x=w308, y=100.0) -> (x*y=w278:dbl)
        n118 = Multiply(x=w266, y=60.0) -> (x*y=w271:dbl)
        n119 = Divide(x=w271, y=w273) -> (x/y=w267:dbl)
        n120 = call-dynamic "Write Multiple Holding Registers.vi"("error in (no error)"=w355, "holding register values"=u16[] [95], "starting address"=u16 60 ("write operation starting address"), "Modbus master in"=w356) -> ("error out"=w351:errorcluster, "Modbus master out"=w350:refnum<class "Modbus Master.lvclass">)  [unwired: 6 in]
        n121 = In Range and Coerce(upper limit=100.0, x=w278, lower limit=0.0) -> (coerced(x)=w275:dbl)  [unwired: 1 out]
        n122 = Add(x=w292, y=61) -> (x+y=w332:i32)
        n123 = Enqueue Element(queue=w313, element=cluster{"DATA":variant, "status":string} {"DATA"=variant, "status"="Set P178"}) -> ()  [unwired: 2 in, 3 out]
        n124 = Multiply(x=327.67, y=w275) -> (x*y=w336:dbl)
        n125 = Multiply(x=w310, y=10.0) -> (x*y=w347:dbl)
        n126 = Multiply(x=w265, y=w320) -> (x*y=w346:dbl)
        n127 = Multiply(x=w286, y=1000.0) -> (x*y=w284:dbl)
        n128 = Multiply(x=w323, y=w320) -> (x*y=w322:dbl)
        n129 = Build Array(w336, w347, w346) -> (w345:dbl[])
        n130 = Build Array(w267, w284) -> (w342:dbl[])
        n131 = Build Array(w322) -> (w321:dbl[])
        n132 = Build Array(w298) -> (w297:enum16{"CW", "CCW"}[])
        n133 = Build Array(w268) -> (w339:dbl[])
        n134 = call-dynamic "Write Multiple Holding Registers.vi"("error in (no error)"=w351, "holding register values"=w345, "starting address"=w332, "Modbus master in"=w350) -> ("error out"=w344:errorcluster, "Modbus master out"=w343:refnum<class "Modbus Master.lvclass">)  [unwired: 6 in]
        n135 = Divide(x=w268, y=2.0) -> (x/y=w282:dbl)
        n136 = Add(x=w292, y=65) -> (x+y=w330:i32)
        n137 = Multiply(x=w282, y=w274) -> (x*y=w281:dbl)
        n138 = Divide(x=w281, y=60.0) -> (x/y=w280:dbl)
        n139 = call-dynamic "Write Multiple Holding Registers.vi"("error in (no error)"=w344, "holding register values"=w342, "starting address"=w330, "Modbus master in"=w343) -> ("error out"=w340:errorcluster, "Modbus master out"=w341:refnum<class "Modbus Master.lvclass">)  [unwired: 6 in]
        n140 = call "Calcola compensaz scorr.vi"("RPM nom"=w274, "#poles"=w268, "Fmax [Hz]"=w280, "Fn [Hz]"=w265) -> ("%Fmax"=w287:dbl)  [unwired: 7 in]
        n141 = Add(x=w292, y=u16 67 ("starting address")) -> (x+y=w328:i32)
        n142 = Multiply(x=327.67, y=w287) -> ()  [unwired: 1 out]
        n143 = call-dynamic "Write Multiple Holding Registers.vi"("error in (no error)"=w340, "holding register values"=w339, "starting address"=w328, "Modbus master in"=w341) -> ("error out"=w327:errorcluster, "Modbus master out"=w326:refnum<class "Modbus Master.lvclass">)  [unwired: 6 in]
        n144 = Add(x=w292, y=71) -> (x+y=w324:i32)
        n145 = call-dynamic "Write Multiple Holding Registers.vi"("error in (no error)"=w327, "holding register values"=w321, "starting address"=w324, "Modbus master in"=w326) -> ("error out"=w294:errorcluster, "Modbus master out"=w296:refnum<class "Modbus Master.lvclass">)  [unwired: 6 in]
        n146 = Build Array(0.0 ("element")) -> (w289:dbl[])
        n147 = Add(x=w292, y=170) -> (x+y=w291:i32)
        n148 = Add(x=76, y=w299) -> (x+y=w304:i32)
        n149 = call-dynamic "Write Multiple Holding Registers.vi"("error in (no error)"=w294, "holding register values"=w289, "starting address"=w291, "Modbus master in"=w296) -> ("error out"=w293:errorcluster, "Modbus master out"=w295:refnum<class "Modbus Master.lvclass">)  [unwired: 6 in]
        n150 = call-dynamic "Write Multiple Holding Registers.vi"("error in (no error)"=w293, "holding register values"=w297, "starting address"=w304, "Modbus master in"=w295) -> ("error out"=w302:errorcluster, "Modbus master out"=w303:refnum<class "Modbus Master.lvclass">)  [unwired: 6 in]
        n151 = flat-sequence {
          tunnel: w302 -> [w359]
          tunnel: w303 -> [w360]
          tunnel: [w360] -> w315
          tunnel: [w359] -> w314
          tunnel: [w362] -> w317
          tunnel: [w361] -> w316
          tunnel: w315 -> [w362]
          tunnel: w314 -> [w361]
          frame #0 {
            n152 = Wait (ms)(milliseconds to wait=u32 500) -> ()  [unwired: 1 out]
          }
          frame #1 {
          }
        }
      }
      frame "Set P178" {
        (unwired) u16[] [] ("register values")
        w410 = T4 0 items=["Table of parameters (P00-P199)", "Table of connections (C00-C99)", "Table of application parameters (E00-E99)", "Table of expanded application parameters (E100-E600)", "Table of internal values (D00-D127)", "Drive state", "Drive alarms", "Alarm enabling", "Speed reference from fieldbus", "Torque limit from fieldbus", "Torque reference from fieldbus", "Mechanical position read", "Logic functions of digital input", "Logic funtction of digital input from serial c.", "logical function of standard digital outputs", "logic function of application digital output", "Table of parameters formats", "Table of connections formats", "Table of monitor and analog outputs values", "Table of application parameters formats", "Table of internal values formats", "Scorta 1", "Scorta 2", "Scorta 3", "Scorta 4", "Scorta 5", "Scorta 6", "Scorta 7", "Scorta 8", "Scorta 9", "Scorta 10"] ("Lista tipi di parametro")
        n153 = call-dynamic "Write Multiple Holding Registers.vi"("error in (no error)"=w369, "holding register values"=u16[] [95], "starting address"=u16 60 ("write operation starting address"), "Modbus master in"=w371) -> ("error out"=w368:errorcluster, "Modbus master out"=w370:refnum<class "Modbus Master.lvclass">)  [unwired: 6 in]
        n154 = call "Indice registri.vi"("Lista tipi di parametro"=w410, "Mappa registri"=w411) -> ("Registro iniziale"=w397:i32)  [unwired: 7 in, 2 out]
        n155 = Add(x=63, y=w397) -> (x+y=w409:i32)
        n156 = Add(x=178, y=w397) -> (x+y=w396:i32)
        n157 = call-dynamic "Read Holding Registers.vi"("error in (no error)"=w368, "number of holding registers"=u16 5, "starting address"=w409, "Modbus master in"=w370) -> ("error out"=w399:errorcluster, "register values"=w407:u16[], "Modbus master out"=w400:refnum<class "Modbus Master.lvclass">)  [unwired: 5 in]
        n158 = Index Array(array=w407) -> (element #1=w406:u16, element #3=w386:u16, element #5=w385:u16)  [unwired: 5 in, 2 out]
        n159 = Divide(x=w406, y=u16 10) -> (x/y=w404:dbl)
        n160 = Divide(x=w385, y=2.0) -> (x/y=w388:dbl)
        n161 = Multiply(x=w386, y=w388) -> (x*y=w390:dbl)
        n162 = Divide(x=w390, y=60.0) -> (x/y=w384:dbl)
        n163 = Flush Queue(queue=w363) -> (queue out=w364:refnum<queue>)  [unwired: 1 in, 2 out]
        n164 = Divide(x=w404, y=w384) -> (x/y=w403:dbl)
        n165 = Multiply(x=100.0, y=w403) -> (x*y=w382:dbl)
        n166 = Enqueue Element(queue=w364, element=cluster{"DATA":variant, "status":string} {"DATA"=variant, "status"="READ"}) -> ()  [unwired: 2 in, 3 out]
        n167 = In Range and Coerce(upper limit=100.0, x=w382, lower limit=0.0) -> (coerced(x)=w381:dbl)  [unwired: 1 out]
        n168 = Multiply(x=100.0, y=40.96) -> (x*y=w377:dbl)
        n169 = To Unsigned Word Integer(number=w377) -> (unsigned 16bit integer=w378:u16)
        n170 = Multiply(x=w381, y=40.96) -> (x*y=w393:dbl)
        n171 = Build Array(w378) -> (w374:u16[])
        n172 = To Unsigned Word Integer(number=w393) -> (unsigned 16bit integer=w392:u16)
        n173 = Build Array(w392) -> (w401:u16[])
        n174 = for {
          N: 20 -> [_]
          tunnel: w401 -> [w429]
          tunnel: w396 -> [w421]
          shift-right: [w426] -> w394
          shift-left: w400 -> [w417]
          shift-right: [w424] -> w395
          shift-left: w399 -> [w420]
          tunnel: w374 -> [w415]
          stop <- w428 stop-if-true
          n175 = Decrement(x=w421) -> (x-1=w418:i32)
          n176 = call-dynamic "Write Multiple Holding Registers.vi"("error in (no error)"=w420, "holding register values"=w415, "starting address"=w418, "Modbus master in"=w417) -> ("error out"=w419:errorcluster, "Modbus master out"=w416:refnum<class "Modbus Master.lvclass">)  [unwired: 6 in]
          n177 = call-dynamic "Write Multiple Holding Registers.vi"("error in (no error)"=w419, "holding register values"=w429, "starting address"=w421, "Modbus master in"=w416) -> ("error out"=w425:errorcluster, "Modbus master out"=w427:refnum<class "Modbus Master.lvclass">)  [unwired: 6 in]
          n178 = Wait (ms)(milliseconds to wait=u32 100) -> ()  [unwired: 1 out]
          n179 = call-dynamic "Read Holding Registers.vi"("error in (no error)"=w425, "number of holding registers"=u16 1, "starting address"=w421, "Modbus master in"=w427) -> ("error out"=w424:errorcluster, "register values"=w422:u16[], "Modbus master out"=w426:refnum<class "Modbus Master.lvclass">)  [unwired: 5 in]
          n180 = Equal?(x=w422, y=w429) -> (x = y?=w428:bool)
        }
      }
      frame "Set F" {
        n181 = Variant To Data(type=T5 {"F [Hz]"=0.0} ("Set inverter"), Variant=w449) -> (data=w447:T5)  [unwired: 1 in, 1 out]
        n182 = Unbundle By Name(w447) -> ("F [Hz]"=w446:dbl)
        n183 = Divide(x=w443, y=u16 2) -> (x/y=w441:dbl)
        n184 = Multiply(x=w446, y=60.0) -> (x*y=w444:dbl)
        n185 = Divide(x=w444, y=w441) -> (x/y=w433:dbl)
        n186 = call-dynamic "Write Multiple Holding Registers.vi"("error in (no error)"=w452, "holding register values"=u16[] [95], "starting address"=u16 60 ("write operation starting address"), "Modbus master in"=w453) -> ("error out"=w456:errorcluster, "Modbus master out"=w455:refnum<class "Modbus Master.lvclass">)  [unwired: 6 in]
        n187 = Divide(x=w433, y=w434) -> (x/y=w440:dbl)
        n188 = Multiply(x=w440, y=100.0) -> (x*y=w438:dbl)
        n189 = Multiply(x=w438, y=163.84) -> (x*y=w436:dbl)
        n190 = Build Array(w436) -> (w435:dbl[])
        n191 = call-dynamic "Write Multiple Holding Registers.vi"("error in (no error)"=w456, "holding register values"=w435, "starting address"=u16 704, "Modbus master in"=w455) -> ("error out"=w450:errorcluster, "Modbus master out"=w451:refnum<class "Modbus Master.lvclass">)  [unwired: 6 in]
      }
      frame "Set Velocità" {
        n192 = Variant To Data(type=0.0, Variant=w474) -> (data=w459:dbl)  [unwired: 1 in, 1 out]
        n193 = call-dynamic "Write Multiple Holding Registers.vi"("error in (no error)"=w477, "holding register values"=u16[] [95], "starting address"=u16 60 ("write operation starting address"), "Modbus master in"=w478) -> ("error out"=w481:errorcluster, "Modbus master out"=w480:refnum<class "Modbus Master.lvclass">)  [unwired: 6 in]
        n194 = Divide(x=w459, y=w466) -> (x/y=w472:dbl)
        n195 = Multiply(x=w472, y=100.0) -> (x*y=w470:dbl)
        n196 = In Range and Coerce(upper limit=100.0, x=w470, lower limit=0.0) -> (coerced(x)=w463:dbl)  [unwired: 1 out]
        n197 = Multiply(x=w463, y=163.84) -> (x*y=w468:dbl)
        n198 = Build Array(w468) -> (w467:dbl[])
        n199 = call-dynamic "Write Multiple Holding Registers.vi"("error in (no error)"=w481, "holding register values"=w467, "starting address"=u16 704, "Modbus master in"=w480) -> ("error out"=w475:errorcluster, "Modbus master out"=w476:refnum<class "Modbus Master.lvclass">)  [unwired: 6 in]
      }
      frame "Run command" {
        w491 = T4 1 items=["Table of parameters (P00-P199)", "Table of connections (C00-C99)", "Table of application parameters (E00-E99)", "Table of expanded application parameters (E100-E600)", "Table of internal values (D00-D127)", "Drive state", "Drive alarms", "Alarm enabling", "Speed reference from fieldbus", "Torque limit from fieldbus", "Torque reference from fieldbus", "Mechanical position read", "Logic functions of digital input", "Logic funtction of digital input from serial c.", "logical function of standard digital outputs", "logic function of application digital output", "Table of parameters formats", "Table of connections formats", "Table of monitor and analog outputs values", "Table of application parameters formats", "Table of internal values formats", "Scorta 1", "Scorta 2", "Scorta 3", "Scorta 4", "Scorta 5", "Scorta 6", "Scorta 7", "Scorta 8", "Scorta 9", "Scorta 10"] ("Lista tipi di parametro")
        n200 = Variant To Data(type=TRUE, Variant=w493) -> (data=w484:bool)  [unwired: 1 in, 1 out]
        n201 = call "Indice registri.vi"("Lista tipi di parametro"=w491, "Mappa registri"=w490) -> ("Registro iniziale"=w489:i32)  [unwired: 7 in, 2 out]
        n202 = Add(x=21, y=w489) -> (x+y=w487:i32)
        n203 = call-dynamic "Write Multiple Holding Registers.vi"("error in (no error)"=w498, "holding register values"=u16[] [95], "starting address"=u16 60 ("write operation starting address"), "Modbus master in"=w499) -> ("error out"=w501:errorcluster, "Modbus master out"=w500:refnum<class "Modbus Master.lvclass">)  [unwired: 6 in]
        n204 = case shown="True" w484 {
          tunnel: w501 -> [w514 w536]
          tunnel: w500 -> [w513 w535]
          tunnel: [w512 w534] -> w497
          tunnel: [w511 w533] -> w496
          tunnel: w484 -> [_ _]
          tunnel: w487 -> [w510 w532]
          frame True {
            # "start attivo sul fronte di salita.\nImposto prima a 0 per resettare lo\nstart nel caso fosse già a 1"
            n205 = flat-sequence {
              tunnel: w514 -> [w520]
              tunnel: w513 -> [w519]
              tunnel: w510 -> [w515]
              tunnel: [w518] -> w509
              tunnel: [w517] -> w508
              tunnel: [w515] -> w504
              tunnel: w509 -> [w524]
              tunnel: w508 -> [w523]
              tunnel: [w524] -> w507
              tunnel: [w523] -> w506
              tunnel: [w521] -> w505
              tunnel: w504 -> [w521]
              tunnel: [w528] -> w511
              tunnel: [w527] -> w512
              tunnel: w507 -> [w530]
              tunnel: w506 -> [w529]
              tunnel: w505 -> [w526]
              frame #0 {
                n206 = call-dynamic "Write Multiple Holding Registers.vi"("error in (no error)"=w520, "holding register values"=u16[] [0], "starting address"=w515, "Modbus master in"=w519) -> ("error out"=w517:errorcluster, "Modbus master out"=w518:refnum<class "Modbus Master.lvclass">)  [unwired: 6 in]
              }
              frame #1 {
                n207 = Wait (ms)(milliseconds to wait=u32 250) -> ()  [unwired: 1 out]
              }
              frame #2 {
                n208 = call-dynamic "Write Multiple Holding Registers.vi"("error in (no error)"=w529, "holding register values"=u16[] [1], "starting address"=w526, "Modbus master in"=w530) -> ("error out"=w528:errorcluster, "Modbus master out"=w527:refnum<class "Modbus Master.lvclass">)  [unwired: 6 in]
              }
            }
          }
          frame False {
            n209 = call-dynamic "Write Multiple Holding Registers.vi"("error in (no error)"=w536, "holding register values"=u16[] [0], "starting address"=w532, "Modbus master in"=w535) -> ("error out"=w533:errorcluster, "Modbus master out"=w534:refnum<class "Modbus Master.lvclass">)  [unwired: 6 in]
          }
        }
      }
      frame "Senso rotazione" {
        w547 = T4 1 items=["Table of parameters (P00-P199)", "Table of connections (C00-C99)", "Table of application parameters (E00-E99)", "Table of expanded application parameters (E100-E600)", "Table of internal values (D00-D127)", "Drive state", "Drive alarms", "Alarm enabling", "Speed reference from fieldbus", "Torque limit from fieldbus", "Torque reference from fieldbus", "Mechanical position read", "Logic functions of digital input", "Logic funtction of digital input from serial c.", "logical function of standard digital outputs", "logic function of application digital output", "Table of parameters formats", "Table of connections formats", "Table of monitor and analog outputs values", "Table of application parameters formats", "Table of internal values formats", "Scorta 1", "Scorta 2", "Scorta 3", "Scorta 4", "Scorta 5", "Scorta 6", "Scorta 7", "Scorta 8", "Scorta 9", "Scorta 10"] ("Lista tipi di parametro")
        n210 = Variant To Data(type=TRUE, Variant=w549) -> (data=w543:bool)  [unwired: 1 in, 1 out]
        n211 = call "Indice registri.vi"("Lista tipi di parametro"=w547, "Mappa registri"=w546) -> ("Registro iniziale"=w545:i32)  [unwired: 7 in, 2 out]
        n212 = call-dynamic "Write Multiple Holding Registers.vi"("error in (no error)"=w554, "holding register values"=u16[] [95], "starting address"=u16 60 ("write operation starting address"), "Modbus master in"=w555) -> ("error out"=w557:errorcluster, "Modbus master out"=w556:refnum<class "Modbus Master.lvclass">)  [unwired: 6 in]
        n213 = Select(t=u16[] [1] ("holding register values"), s=w543, f=u16[] [0] ("holding register values")) -> (s? t:f=w539:u16[])
        n214 = Add(x=76, y=w545) -> (x+y=w542:i32)
        n215 = call-dynamic "Write Multiple Holding Registers.vi"("error in (no error)"=w557, "holding register values"=w539, "starting address"=w542, "Modbus master in"=w556) -> ("error out"=w552:errorcluster, "Modbus master out"=w553:refnum<class "Modbus Master.lvclass">)  [unwired: 6 in]
      }
      frame "Reset allarmi" {
        w574 = T4 1 items=["Table of parameters (P00-P199)", "Table of connections (C00-C99)", "Table of application parameters (E00-E99)", "Table of expanded application parameters (E100-E600)", "Table of internal values (D00-D127)", "Drive state", "Drive alarms", "Alarm enabling", "Speed reference from fieldbus", "Torque limit from fieldbus", "Torque reference from fieldbus", "Mechanical position read", "Logic functions of digital input", "Logic funtction of digital input from serial c.", "logical function of standard digital outputs", "logic function of application digital output", "Table of parameters formats", "Table of connections formats", "Table of monitor and analog outputs values", "Table of application parameters formats", "Table of internal values formats", "Scorta 1", "Scorta 2", "Scorta 3", "Scorta 4", "Scorta 5", "Scorta 6", "Scorta 7", "Scorta 8", "Scorta 9", "Scorta 10"] ("Lista tipi di parametro")
        n216 = call "Indice registri.vi"("Lista tipi di parametro"=w574, "Mappa registri"=w573) -> ("Registro iniziale"=w572:i32)  [unwired: 7 in, 2 out]
        n217 = Add(x=w572, y=30) -> (x+y=w562:i32)
        n218 = flat-sequence {
          tunnel: w562 -> [w581]
          tunnel: w570 -> [w580]
          tunnel: [w579] -> w568
          tunnel: w566 -> [w578]
          tunnel: [w577] -> w564
          tunnel: [w584] -> w569
          tunnel: w568 -> [w584]
          tunnel: [w583] -> w565
          tunnel: w564 -> [w583]
          tunnel: w569 -> [w590]
          tunnel: [w589] -> w567
          tunnel: w565 -> [w588]
          tunnel: [w587] -> w563
          tunnel: w562 -> [w586]
          frame #0 {
            n219 = call-dynamic "Write Multiple Holding Registers.vi"("error in (no error)"=w578, "holding register values"=u16[] [1], "starting address"=w581, "Modbus master in"=w580) -> ("error out"=w577:errorcluster, "Modbus master out"=w579:refnum<class "Modbus Master.lvclass">)  [unwired: 6 in]
          }
          frame #1 {
            n220 = Wait (ms)(milliseconds to wait=u32 500) -> ()  [unwired: 1 out]
          }
          frame #2 {
            n221 = call-dynamic "Write Multiple Holding Registers.vi"("error in (no error)"=w588, "holding register values"=u16[] [0], "starting address"=w586, "Modbus master in"=w590) -> ("error out"=w587:errorcluster, "Modbus master out"=w589:refnum<class "Modbus Master.lvclass">)  [unwired: 6 in]
          }
        }
      }
      frame "Close modbus" {
        n222 = flat-sequence {
          tunnel: w598 -> [w599]
          frame #0 {
            n223 = call-dynamic "Close.vi"("Modbus master in"=w599) -> ()  [unwired: 10 in, 1 out]
          }
          frame #1 {
            n224 = Wait (ms)(milliseconds to wait=u32 1500) -> ()  [unwired: 1 out]
          }
        }
        n225 = Enqueue Element(queue=w596, element=cluster{"DATA":variant, "status":string} {"DATA"=variant, "status"="Initialize"}) -> ()  [unwired: 2 in, 3 out]
      }
      frame "Stop" {
        n226 = call-dynamic "Close.vi"("error in (no error)"=w605, "Modbus master in"=w606) -> ()  [unwired: 9 in, 1 out]
      }
      frame "Scelta inverter" {
        n227 = Variant To Data(type=u8 0 ("unit ID"), Variant=w617) -> (data=w613:u8)  [unwired: 1 in, 1 out]
        "id" <- w613
        n228 = Not Equal?(x=w613, y=u8 3) -> (x != y?=w611:bool)
        n229 = Not Equal To 0?(x=w613) -> (x != 0?=w610:bool)
        n230 = And(x=w610, y=w611) -> (x .and. y?=w609:bool)
        n231 = case shown="True" w609 {
          tunnel: w619 -> [w626 w630]
          tunnel: [w626 w639] -> w618
          tunnel: w613 -> [_ w627]
          tunnel: w615 -> [w624 w637]
          tunnel: w608 -> [_ w628]
          frame False {
            n232 = Flush Queue(queue=w624) -> (queue out=w623:refnum<queue>)  [unwired: 1 in, 2 out]
            n233 = Enqueue Element(queue=w623, element=cluster{"DATA":variant, "status":string} {"DATA"=variant, "status"="IDLE"}) -> ()  [unwired: 2 in, 3 out]
          }
          frame True {
            w632 = u16 0 items=["None", "XON/XOFF", "RTS/CTS", "XON/XOFF & RTS/CTS", "DTR/DSR", "XON/XOFF & DTR/DSR"] ("flow control (None)")
            w633 = u16 0 items=["None", "Odd", "Even"] ("parity (Even)")
            n234 = call-dynamic "Close.vi"("Modbus master in"=w630) -> ("error out"=w635:errorcluster)  [unwired: 10 in]
            n235 = call <vilib>:"Clear Errors.vi"("error in (no error)"=w635) -> ("error out"=w636:errorcluster)  [unwired: 5 in, 1 out]
            n236 = call-poly <vilib>:"Create Master Instance.vi"("flow control (None)"=w632, "serial type"=enum16{"RTU", "ASCII"}."RTU", "parity (Even)"=w633, "unit ID"=w627, "error in (no error)"=w636, "baud rate (9600)"=u32 19200, "VISA resource name"=w628) -> ("serial master instance"=w629:refnum<class "Modbus Master.lvclass">)  [unwired: 3 in, 1 out]
            n237 = property class="Modbus Master"(reference=w629, "Data Access:Unit ID"=w627) -> (reference out=w639:refnum<class "Modbus Master.lvclass">)  [unwired: 1 in, 1 out]
            n238 = Enqueue Element(queue=w637, element=cluster{"DATA":variant, "status":string} {"DATA"=variant, "status"="READ"}) -> ()  [unwired: 2 in, 3 out]
          }
        }
        n239 = property class="Bool (strict)"(reference=w614, "Visible"=w609) -> ()  [unwired: 1 in, 2 out]
      }
      frame "IDLE" {
      }
    }
    "Numeric" <- w70
  }
  n240 = call-dynamic "Close.vi"("error in (no error)"=w27, "Modbus master in"=w26) -> ()  [unwired: 9 in, 1 out]
